vi "APC_9049_keyCA50.vi"(0 "CA50":dbl[](array[numeric])) -> ()   [LabVIEW 2020]
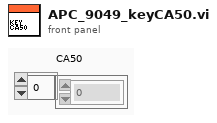
[diagram p1: front panel]
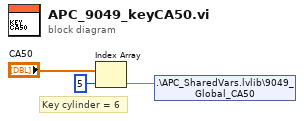
[diagram p0: block diagram]
diagram:
  # "Key cylinder = 6"
  n1 = Index Array(array="CA50", index=5) -> (element=w3:dbl)
  n2 = shared-variable ".\\APC_SharedVars.lvlib\\9049_Global_CA50"(w3) -> ()  [unwired: 1 in, 1 out]
